vi "Write Time Out Ref.vi"(8 "error in (no error)":errorcluster, 10 "Numeric":i32, 11 "Data Logger in":refnum<class "Data Logger.lvclass">) -> (0 "error out":errorcluster, 3 "Data Logger out":refnum<class "Data Logger.lvclass">)   [LabVIEW 2013, in "Data Logger.lvlib" / "Data Logger.lvclass"]
uses:
  Data Logger.lvclass
  Data Logger.lvclass/Data Logger.ctl
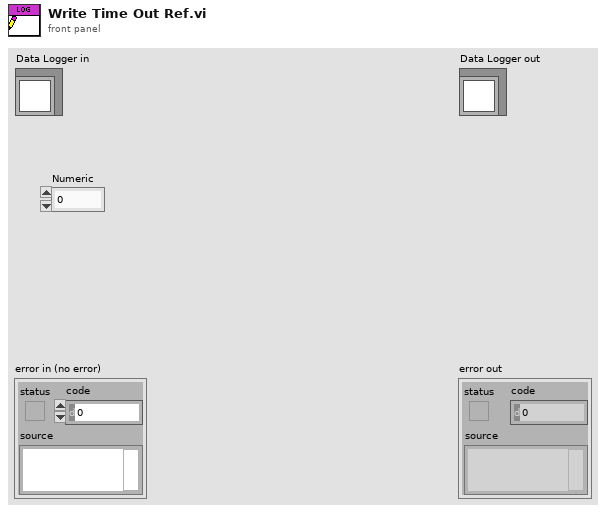
[diagram p1: front panel]
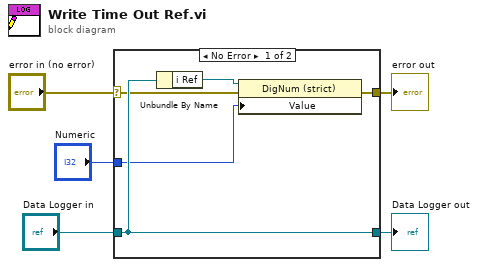
[diagram p0: block diagram]
diagram:
  n1 = case shown="No Error" "error in (no error)" {
    selector: "error in (no error)" -> [w7 w11]
    tunnel: [w6 w11] -> w4
    tunnel: [w10 w12] -> w2
    tunnel: "Data Logger in" -> [w10 w12]
    tunnel: "Numeric" -> [w8 _]
    frame No Error {
      n2 = Unbundle By Name(w10) -> ("i Ref"=w9:refnum<vi>)
      n3 = property class="DigNum (strict)"(reference=w9, error in=w7, "Value"=w8) -> (error out=w6:errorcluster)  [unwired: 1 out]
    }
    frame Error {
    }
  }
  "error out" <- w4
  "Data Logger out" <- w2
